vi "Init Tx - UDP Connection.vi"(8 "error in (no error)":errorcluster, 11 "Tx Loop Data in":T1) -> (0 "error out":errorcluster, 3 "Tx Loop Data out":T1)   [LabVIEW 2016, in "UDP-Custom-Device Engine.lvlib"]
uses:
  UDP-Custom-Device Engine.lvlib
  Types/Engine - Tx Loop Data.ctl
  <vilib>/NI Veristand/VeriStand Data/Byte Buffer/Byte Buffer.lvclass
  Types/Engine - General Resources.ctl
  <vilib>/NI Veristand/VeriStand Data/Typedefs/Typedefs.Data Types.ctl
  Shared/Types/Shared - Duplex Settings.ctl
  Shared/Types/Shared - Header Details.ctl
  Types/Engine - Data Conversion Config.ctl
  <vilib>/NI Veristand/VeriStand Data/Byte Buffer/Byte Buffer.Mapping.ctl
  Types/Engine - Tx Runtime Resources.ctl
  Shared/Types/Shared - Transmit Flag Options.ctl
  Types/Engine - Execution Config.ctl
  Shared/Types/Shared - Thread Management.ctl
  Types/Engine - Tx Echo Resources.ctl
  Shared/Types/Shared - Transmit Echo Options.ctl
  Types/Engine - Tx Channel Refs.ctl
  <vilib>/NI/NIVS Inline Async API/_Data Access Engine/Data Access Engine/Types/Read.DVR.ctl
  <vilib>/NI/NIVS Inline Async API/_Data Access Engine/Access Type Classes/Read/Read.lvclass
  <vilib>/NI/NIVS Inline Async API/_Data Access Engine/Data Access Engine/Types/Write.DVR.ctl
  <vilib>/NI/NIVS Inline Async API/_Data Access Engine/Access Type Classes/Write/Write.lvclass
  Types/Engine - Debug Resources.ctl
  <vilib>/Utility/tcp.llb/UDP Multicast Write-Only Open.vi
  <vilib>/NI/NIVS Inline Async API/_Data Access Engine/Data Access Engine/Data Access Engine.lvclass
  <vilib>/NI Veristand/VeriStand Data/VeriStand Data.lvlib
  Shared/UDP-Custom-Device Shared.lvlib
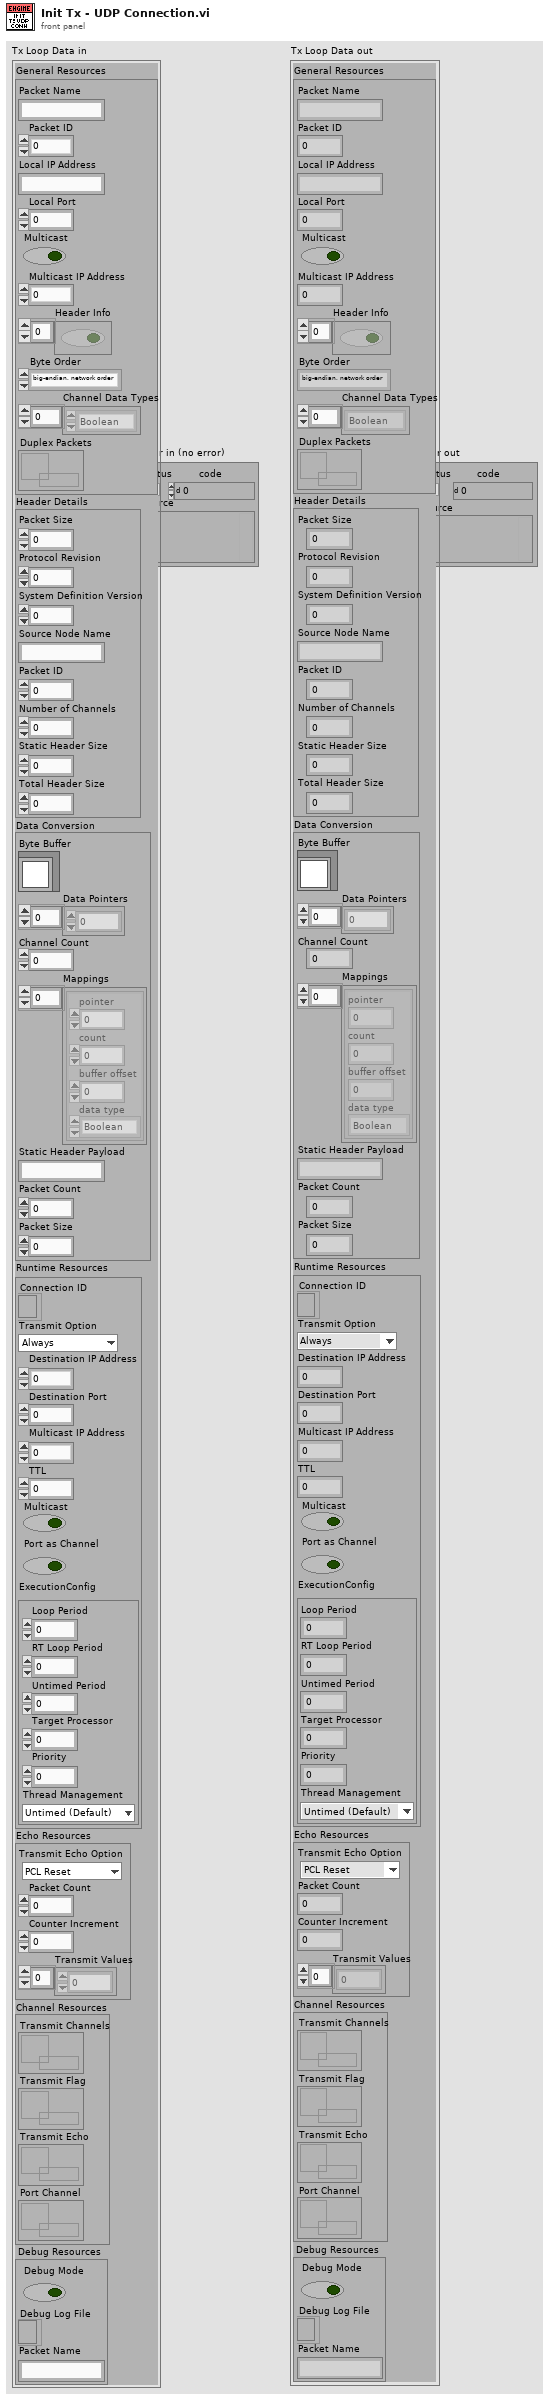
[diagram p1: front panel]
types:
  T1 = typedef "UDP-Custom-Device Engine.lvlib/Engine - Tx Loop Data.ctl" = cluster{"General Resources":T2, "Header Details":T4, "Data Conversion":T5, "Runtime Resources":T7, "Echo Resources":T11, "Channel Resources":T13, "Debug Resources":T16}
  T2 = typedef "UDP-Custom-Device Engine.lvlib/Engine - General Resources.ctl" = cluster{"Packet Name":string, "Packet ID":i32, "Local IP Address":string, "Local Port":i32, "Multicast":bool, "Multicast IP Address":u32, "Header Info":bool[], "Byte Order":enum16{"big-endian, network order", "native, host order", "little-endian"}, "Channel Data Types":T3[], "Duplex Packets":refnum<data-value>}
  T3 = typedef "VeriStand Data.lvlib/Typedefs.Data Types.ctl" = enum16{"Boolean", "Single", "Double", "I8", "I16", "I32", "I64", "U8", "U16", "U32", "U64"}
  T4 = typedef "UDP-Custom-Device Shared.lvlib/Shared - Header Details.ctl" = cluster{"Packet Size":u16, "Protocol Revision":u8, "System Definition Version":u64, "Source Node Name":string, "Packet ID":u32, "Number of Channels":u32, "Static Header Size":u16, "Total Header Size":u16}
  T5 = typedef "UDP-Custom-Device Engine.lvlib/Engine - Data Conversion Config.ctl" = cluster{"Byte Buffer":refnum<class "Byte Buffer.lvclass">, "Data Pointers":u64[], "Channel Count":i32, "Mappings":T6[], "Static Header Payload":string, "Packet Count":dbl, "Packet Size":i32}
  T6 = typedef "VeriStand Data.lvlib/Byte Buffer.lvclass/Byte Buffer.Mapping.ctl" = cluster{"pointer":u64, "count":i64, "buffer offset":u64, "data type":T3}
  T7 = typedef "UDP-Custom-Device Engine.lvlib/Engine - Tx Runtime Resources.ctl" = cluster{"Connection ID":refnum<k16>, "Transmit Option":T8, "Destination IP Address":u32, "Destination Port":u16, "Multicast IP Address":u32, "TTL":u16, "Multicast":bool, "Port as Channel":bool, "ExecutionConfig":T9}
  T8 = typedef "UDP-Custom-Device Shared.lvlib/Shared - Transmit Flag Options.ctl" = enum16{"Always", "One-Shot", "Toggle"}
  T9 = typedef "UDP-Custom-Device Engine.lvlib/Engine - Execution Config.ctl" = cluster{"Loop Period":i64, "RT Loop Period":i64, "Untimed Period":u32, "Target Processor":i32, "Priority":i32, "Thread Management":T10}
  T10 = typedef "UDP-Custom-Device Shared.lvlib/Shared - Thread Management.ctl" = enum16{"Untimed (Default)", "Timed (High Priority)"}
  T11 = typedef "UDP-Custom-Device Engine.lvlib/Engine - Tx Echo Resources.ctl" = cluster{"Transmit Echo Option":T12, "Packet Count":dbl, "Counter Increment":dbl, "Transmit Values":dbl[]}
  T12 = typedef "UDP-Custom-Device Shared.lvlib/Shared - Transmit Echo Options.ctl" = enum16{"PCL Reset", "Counter", "Mirror"}
  T13 = typedef "UDP-Custom-Device Engine.lvlib/Engine - Tx Channel Refs.ctl" = cluster{"Transmit Channels":T14, "Transmit Flag":T14, "Transmit Echo":T15, "Port Channel":T14}
  T14 = typedef "Data Access Engine.lvlib/Data Access Engine.lvclass/Read.DVR.ctl" = refnum<data-value>
  T15 = typedef "Data Access Engine.lvlib/Data Access Engine.lvclass/Write.DVR.ctl" = refnum<data-value>
  T16 = typedef "UDP-Custom-Device Engine.lvlib/Engine - Debug Resources.ctl" = cluster{"Debug Mode":bool, "Debug Log File":refnum<file>, "Packet Name":string}
  T17 = typedef "UDP-Custom-Device Shared.lvlib/Shared - Duplex Settings.ctl" = cluster{"Transmit Packet ID":i32, "Receive Packet ID":i32, "Multicast":bool, "Multicast Address":string, "IP Address":string, "Port":u16, "TTL":u16, "Duplex Connection":refnum<k16>}
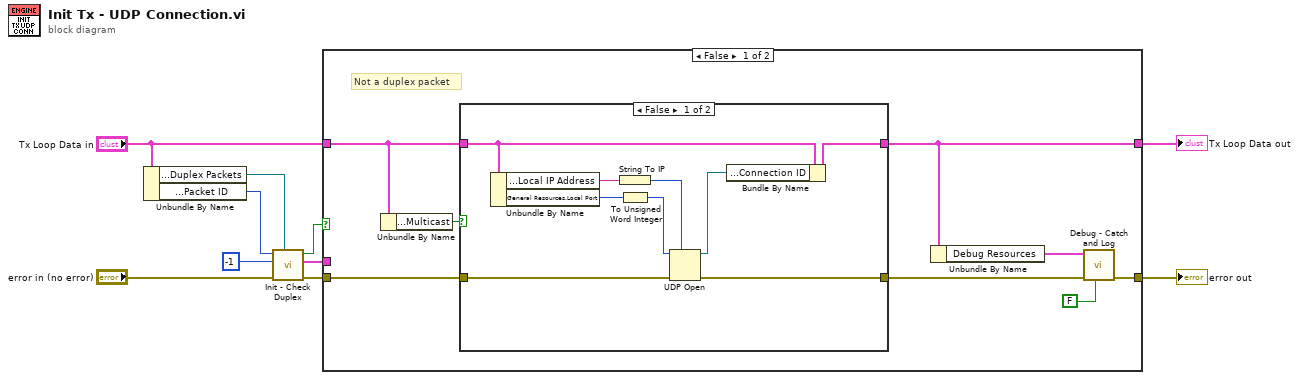
[diagram p0: block diagram]
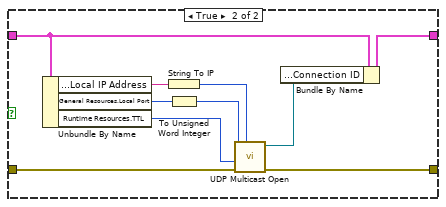
[diagram p2: hidden frame]
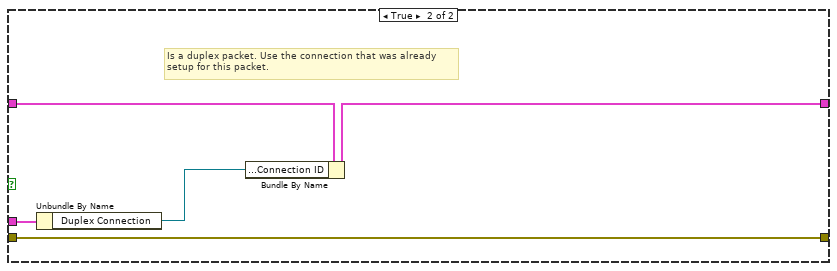
[diagram p3: hidden frame]
diagram:
  n1 = Unbundle By Name("Tx Loop Data in") -> ("General Resources.Duplex Packets"=w8:refnum<data-value>, "General Resources.Packet ID"=w7:i32)
  n2 = call "Init - Check Duplex.vi"("Duplex Packets"=w8, "error in (no error)"="error in (no error)", "Receive Packet ID"=-1, "Transmit Packet ID"=w7) -> ("error out"=w4:errorcluster, "Duplex Settings"=w3:T17, "Is Duplex?"=w2:bool)  [unwired: 5 in]
  n3 = case shown="False" w2 {
    tunnel: w4 -> [w18 w40]
    tunnel: [w15 w40] -> w10
    tunnel: [w12 w38] -> w9
    tunnel: "Tx Loop Data in" -> [w17 w39]
    tunnel: w3 -> [_ w41]
    frame False {
      # "Not a duplex packet"
      n4 = Unbundle By Name(w17) -> ("Runtime Resources.Multicast"=w16:bool)
      n5 = case shown="False" w16 {
        tunnel: w18 -> [w27 w37]
        tunnel: [w26 w36] -> w14
        tunnel: w17 -> [w23 w35]
        tunnel: [w22 w34] -> w12
        frame False {
          n6 = Unbundle By Name(w23) -> ("General Resources.Local IP Address"=w20:string, "General Resources.Local Port"=w25:i32)
          n7 = String To IP(1:w20) -> (0:w19:u32)
          n8 = To Unsigned Word Integer(number=w25) -> (unsigned 16bit integer=w21:u16)
          n9 = UDP Open(7:w19, 8:w27, 11:w21) -> (port=w24:refnum<k16>, 0:w26:errorcluster)  [unwired: 2 in, 1 out]
          n10 = Bundle By Name(cluster=w23, "Runtime Resources.Connection ID"=w24) -> (w22:T1)
        }
        frame True {
          n11 = Unbundle By Name(w35) -> ("General Resources.Local IP Address"=w32:string, "General Resources.Local Port"=w30:i32, "Runtime Resources.TTL"=w28:u16)
          n12 = String To IP(1:w32) -> (0:w31:u32)
          n13 = To Unsigned Word Integer(number=w30) -> (unsigned 16bit integer=w29:u16)
          n14 = call-poly <vilib>:"UDP Multicast Open.vi"("net address"=w31, "error in (no error)"=w37, "time-to-live (1)"=w28, "port"=w29) -> ("error out"=w36:errorcluster, "connection ID"=w33:refnum<k16>)  [unwired: 6 in]
          n15 = Bundle By Name(cluster=w35, "Runtime Resources.Connection ID"=w33) -> (w34:T1)
        }
      }
      n16 = Unbundle By Name(w12) -> ("Debug Resources"=w11:T16)
      n17 = call "Debug - Catch and Log.vi"("Clear Error?"=FALSE, "error in (no error)"=w14, "Debug Resources"=w11) -> ("error out"=w15:errorcluster)  [unwired: 8 in]
    }
    frame True {
      # "Is a duplex packet. Use the connection that was already\nsetup for this packet."
      n18 = Unbundle By Name(w41) -> ("Duplex Connection"=w42:refnum<k16>)
      n19 = Bundle By Name(cluster=w39, "Runtime Resources.Connection ID"=w42) -> (w38:T1)
    }
  }
  "error out" <- w10
  "Tx Loop Data out" <- w9
